vi "强度图.vi"() -> ()   [LabVIEW 2010]
panel:
  in  "颜色数据":i16[][](array[numeric])=[[50, 0, 0, 0], [0, 50, 0, 100], [250, 250, 50, 250], [0, 100, 0, 50], [100, 0, 0, 0]]
  out "强度图表":i16[][](graph)
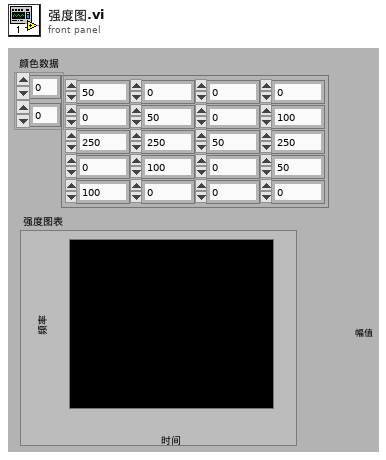
[diagram p1: front panel]
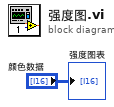
[diagram p0: block diagram]
diagram:
  "强度图表" <- "颜色数据"
